vi "Grade VIA Results.vi"(6 "Grade Per Ranking? (T)":bool=TRUE, 7 "Repo Root":path, 8 "Error in":errorcluster caption="Error in (no error)", 10 "Ranking Thresholds":T1={"High"=100.0, "Normal"=90.0, "Low"=80.0}, 11 "VIAResult":T10 {"Test Config Data"."Test Ranking" items=["Low", "Normal", "High"]}) -> (0 "Error out":errorcluster, 1 "Pass?":bool, 2 "Individual VI Results":string, 3 "VIA+ Results":string)   [LabVIEW 2023, in "VIA Results Handling.lvlib"]
doc: "Takes in VIA Results, Thresholds, Root Directory to determine pass/fail.\n\nOption to choose to grade Per Ranking or Per VI."
uses:
  VIA Results Handling.lvlib
  <vilib>/addons/analyzer/_analyzerctrls.llb/VIAnCtl Results.ctl
  <vilib>/addons/analyzer/_analyzerctrls.llb/VIAnCtl ResultsData (index).ctl
  <vilib>/addons/analyzer/_analyzerctrls.llb/VIAnCtl ResultStatus.ctl
  <vilib>/addons/analyzer/_vianresshared.llb/VIAnRes Parsed Results Data (by VI).ctl
  <vilib>/addons/analyzer/_vianresshared.llb/VIAnRes Parsed Results Data (by Test).ctl
  <vilib>/addons/analyzer/_analyzerctrls.llb/VIAnCtl Test Config Data.ctl
  <vilib>/addons/analyzer/_analyzerctrls.llb/VIAnCtl TestRanking.ctl
  <vilib>/addons/analyzer/_analyzerctrls.llb/VIAnCtl Config Control Value.ctl
  Ranking Thresholds.ctl
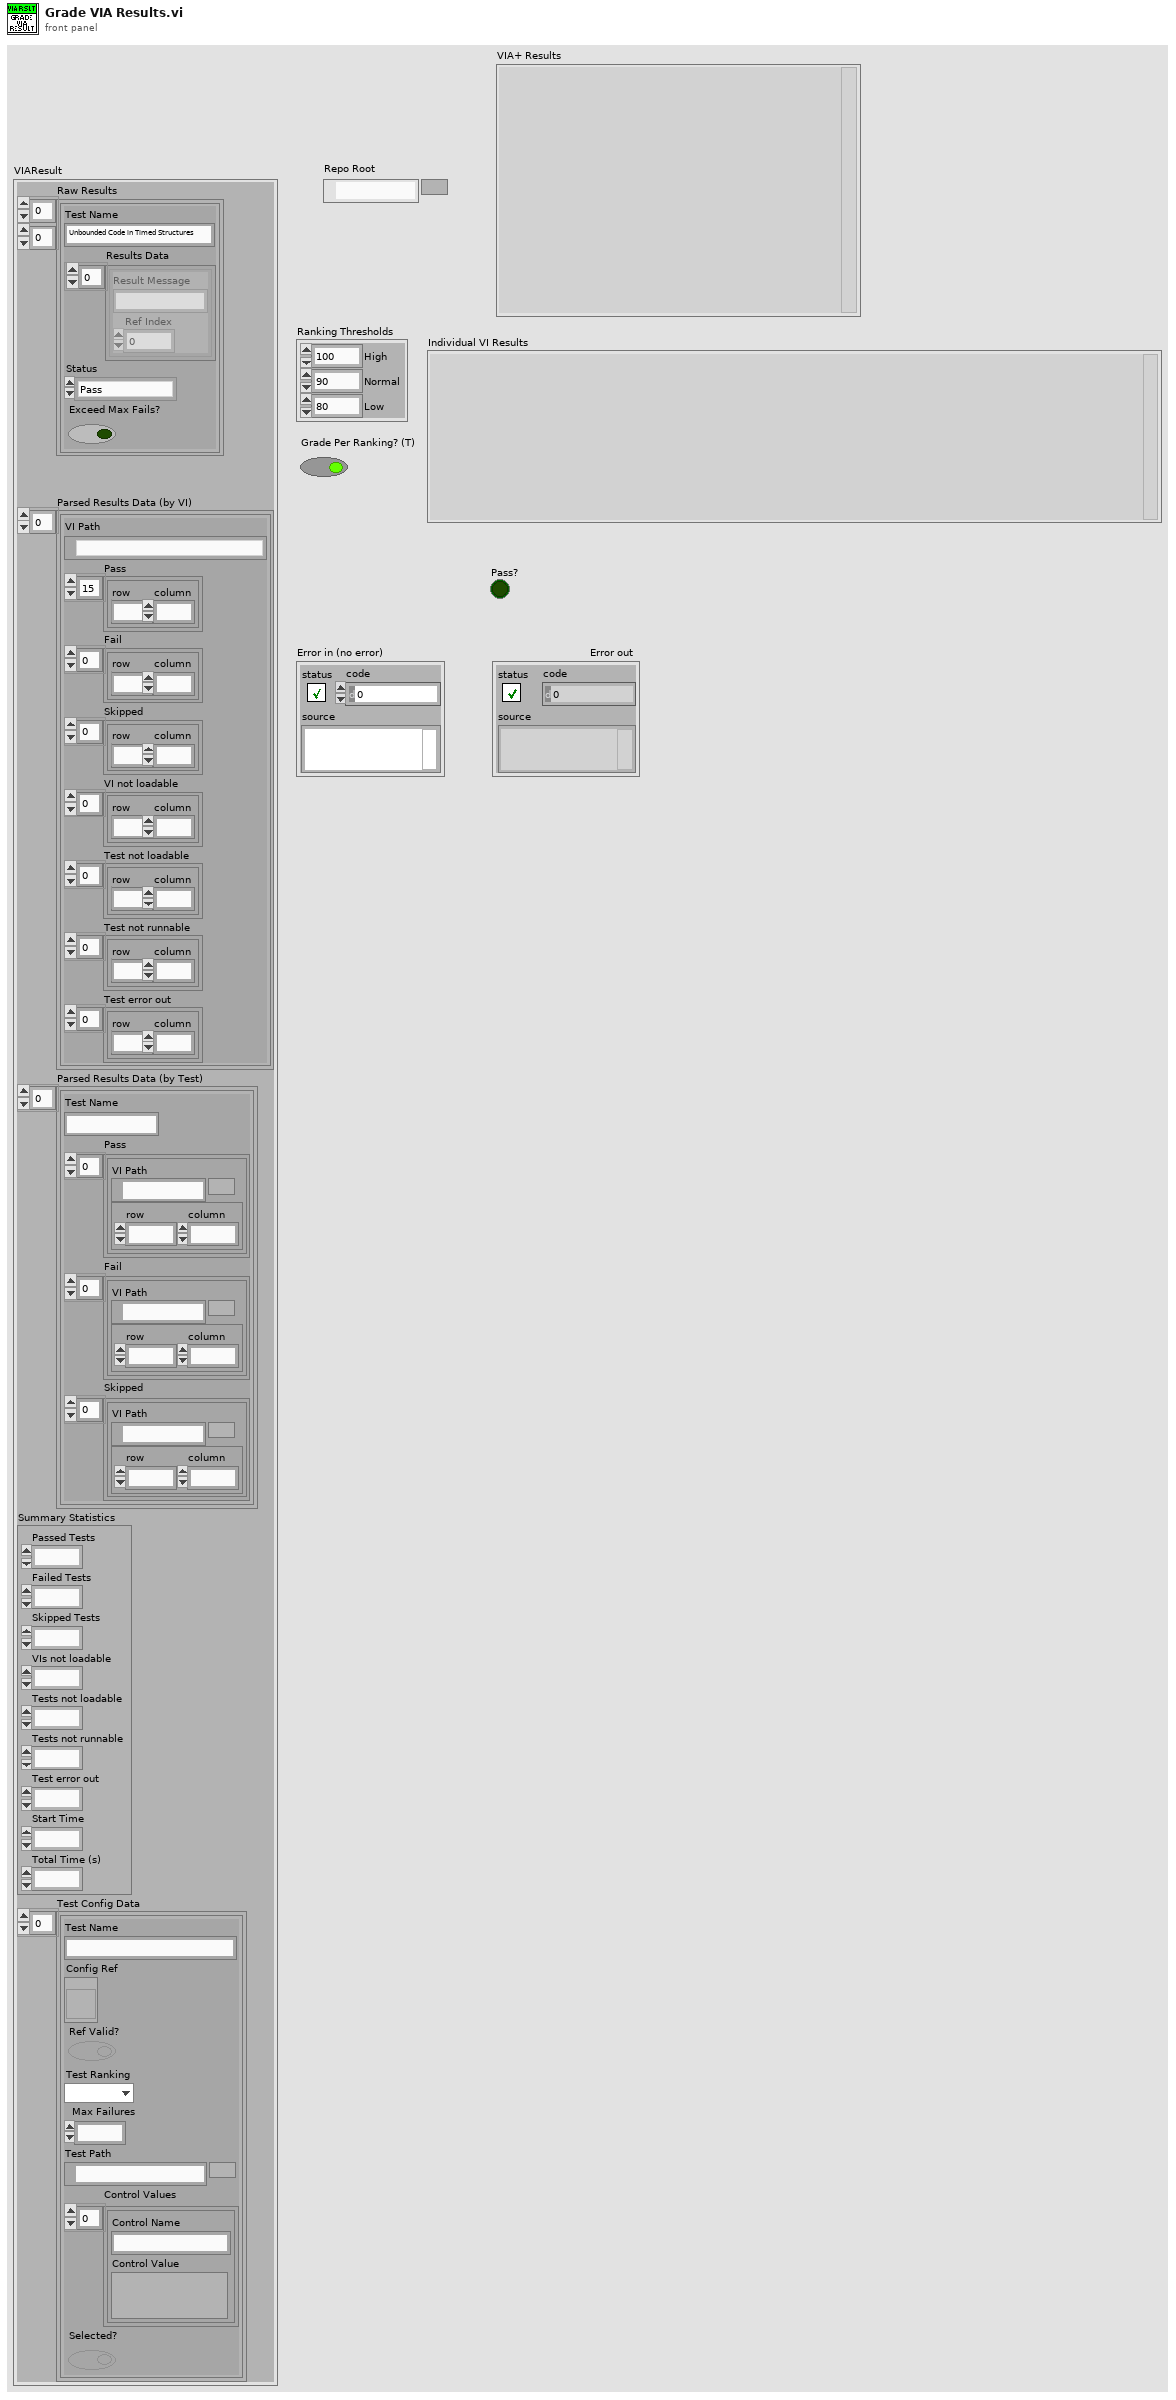
[diagram p1: front panel]
types:
  T1 = typedef "VIA Results Handling.lvlib/Ranking Thresholds.ctl" = cluster{"High":dbl, "Normal":dbl, "Low":dbl}
  T2 = typedef "VIAnCtl Results.ctl" = cluster{"Test Name":string, "Results Data":T3[], "Status":T4, "Exceed Max Fails?":bool}
  T3 = typedef "VIAnCtl ResultsData (index).ctl" = cluster{"Result Message":string, "Ref Index":i32}
  T4 = typedef "VIAnCtl ResultStatus.ctl" = enum16{"Pass", "Fail", "Skipped", "VI not loadable", "Test not loadable", "Test not runnable", "Test error out"}
  T5 = typedef "VIAnRes Parsed Results Data (by VI).ctl" = cluster{"VI Path":path, "Pass":cluster{"row":i32, "column":i32}[], "Fail":cluster{"row":i32, "column":i32}[], "Skipped":cluster{"row":i32, "column":i32}[], "VI not loadable":cluster{"row":i32, "column":i32}[], "Test not loadable":cluster{"row":i32, "column":i32}[], "Test not runnable":cluster{"row":i32, "column":i32}[], "Test error out":cluster{"row":i32, "column":i32}[]}
  T6 = typedef "VIAnRes Parsed Results Data (by Test).ctl" = cluster{"Test Name":string, "Pass":cluster{"VI Path":path, "index":cluster{"row":i32, "column":i32}}[], "Fail":cluster{"VI Path":path, "index":cluster{"row":i32, "column":i32}}[], "Skipped":cluster{"VI Path":path, "index":cluster{"row":i32, "column":i32}}[]}
  T7 = typedef "VIAnCtl Test Config Data.ctl" = cluster{"Test Name":string, "Config Ref":refnum<vi>, "Ref Valid?":bool, "Test Ranking":T8, "Max Failures":u32, "Test Path":path, "Control Values":T9[], "Selected?":bool}
  T8 = typedef "VIAnCtl TestRanking.ctl" = u16
  T9 = typedef "VIAnCtl Config Control Value.ctl" = cluster{"Control Name":string, "Control Value":variant}
  T10 = cluster{"Raw Results":T2[][], "Parsed Results Data (by VI)":T5[], "Parsed Results Data (by Test)":T6[], "Summary Statistics":cluster{"Passed Tests":i32, "Failed Tests":i32, "Skipped Tests":i32, "VIs not loadable":i32, "Tests not loadable":i32, "Tests not runnable":i32, "Test error out":i32, "Start Time":u32, "Total Time (s)":dbl}, "Test Config Data":T7[]}
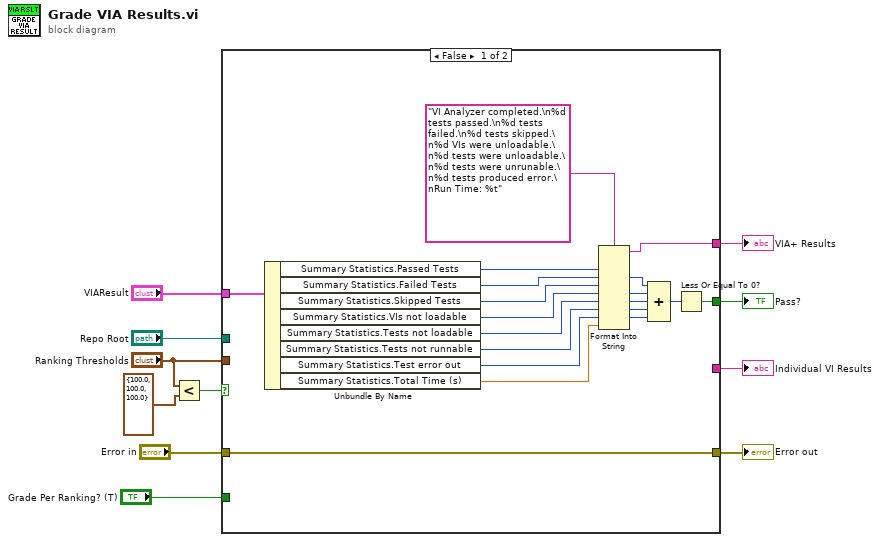
[diagram p0: block diagram]
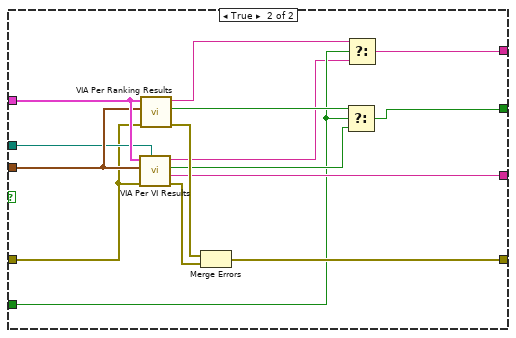
[diagram p2: hidden frame]
diagram:
  n1 = Less?(x="Ranking Thresholds", y=T1 {"High"=100.0, "Normal"=100.0, "Low"=100.0}) -> (x < y?=w4:bool)
  n2 = case shown="False" w4 {
    tunnel: "VIAResult" -> [w16 w40]
    tunnel: "Ranking Thresholds" -> [_ w39]
    tunnel: [w13 w26] -> w10
    tunnel: "Repo Root" -> [_ w38]
    tunnel: [w14 w31] -> w8
    tunnel: "Error in" -> [w12 w37]
    tunnel: [w12 w36] -> w6
    tunnel: "Grade Per Ranking? (T)" -> [_ w29]
    tunnel: [_ w30] -> w1
    frame False {
      n3 = Unbundle By Name(w16) -> ("Summary Statistics.Passed Tests"=w23:i32, "Summary Statistics.Failed Tests"=w21:i32, "Summary Statistics.Skipped Tests"=w24:i32, "Summary Statistics.VIs not loadable"=w20:i32, "Summary Statistics.Tests not loadable"=w19:i32, "Summary Statistics.Tests not runnable"=w18:i32, "Summary Statistics.Test error out"=w17:i32, "Summary Statistics.Total Time (s)"=w25:dbl)
      n4 = Format Into String(format string="VI Analyzer completed.\n%d tests passed.\n%d tests failed.\n%d tests skipped.\n%d VIs were unloadable.\n%d tests were unloadable.\n%d tests were unrunable.\n%d tests produced error.\nRun Time: %t", w23, w21, w24, w20, w19, w18, w17, w25) -> (resulting string=w13:string)  [unwired: 2 in, 1 out]
      n5 = Compound Arithmetic op=ADD(w21, w20, w19, w18, w17) -> (w22:i32)
      n6 = Less Or Equal To 0?(x=w22) -> (x <= 0?=w14:bool)
    }
    frame True {
      n7 = call "VIA Per VI Results.vi"("Root Dir"=w38, "Error in"=w37, "Ranking Thresholds"=w39, "VIAResult"=w40) -> ("Error out"=w34:errorcluster, "Per VI Ranking CSV String"=w30:string, "Pass?"=w33:bool, "Per VI Results String"=w28:string)  [unwired: 4 in]
      n8 = call "VIA Per Ranking Results.vi"("error in (no error)"=w37, "Ranking Thresholds"=w39, "VIAResult"=w40) -> ("error out"=w35:errorcluster, "Pass?"=w32:bool, "Per Ranking Results String"=w27:string)  [unwired: 6 in]
      n9 = Merge Errors(w35, w34) -> (w36:errorcluster)
      n10 = Select(t=w32, s=w29, f=w33) -> (s? t:f=w31:bool)
      n11 = Select(t=w27, s=w29, f=w28) -> (s? t:f=w26:string)
    }
  }
  "Error out" <- w6
  "VIA+ Results" <- w10
  "Individual VI Results" <- w1
  "Pass?" <- w8
